vi "u0v0.vi"(10 "Delta^2":cdb, 11 "(E-iG)^2":cdb[](array[numeric])) -> (1 "v0^2":dbl[](array[numeric]), 2 "u0^2":dbl[](array[numeric]), 3 "(E - i * G)^2 - Delta^2":cdb[](array[numeric]))   [LabVIEW 2021]
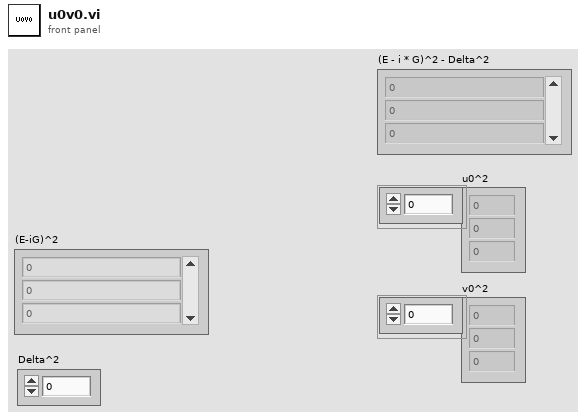
[diagram p1: front panel]
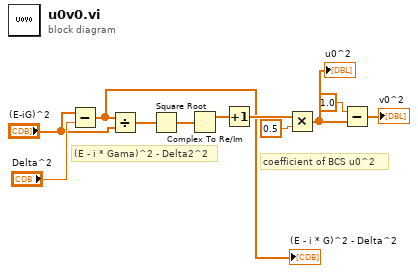
[diagram p0: block diagram]
diagram:
  # "coefficient of BCS u0^2"
  # "(E - i * Gama)^2 - Delta2^2"
  n1 = Subtract(x="(E-iG)^2", y="Delta^2") -> (x-y=w1:cdb[])
  "(E - i * G)^2 - Delta^2" <- w1
  n2 = Divide(x=w1, y="(E-iG)^2") -> (x/y=w5:cdb[])
  n3 = Square Root(x=w5) -> (sqrt(x)=w4:cdb[])
  n4 = Complex To Re/Im(x + iy=w4) -> (x=w7:dbl[])  [unwired: 1 out]
  n5 = Increment(x=w7) -> (x+1=w6:dbl[])
  n6 = Multiply(x=w6, y=0.5) -> (x*y=w3:dbl[])
  "u0^2" <- w3
  n7 = Subtract(x=1.0, y=w3) -> (x-y=→"v0^2":dbl[])
